vi "subVI PID.vi"(5 "PID gains":T1={"proportional gain (Kc)"=1.0, "integral time (Ti, s)"=0.01, "derivative time (Td, s)"=0.0} {"derivative time (Td, s)" format="%.3f"; "integral time (Ti, s)" format="%.3f"; "proportional gain (Kc)" format="%.3f"}, 6 "input":dbl, 7 "output range":cluster{"output high":dbl, "output low":dbl}={"output high"=100.0, "output low"=-100.0} {"output low" format="%.2f"; "output high" format="%.2f"}, 8 "reinitialize? (F)":bool, 9 "dt (s)":dbl=-1.0 format="%.3f", 10 "process variable":dbl format="%.2f", 11 "setpoint":dbl format="%.2f") -> (0 "dt out (s)":dbl format="%.3f", 3 "output":dbl format="%.2f")   [LabVIEW 2017]
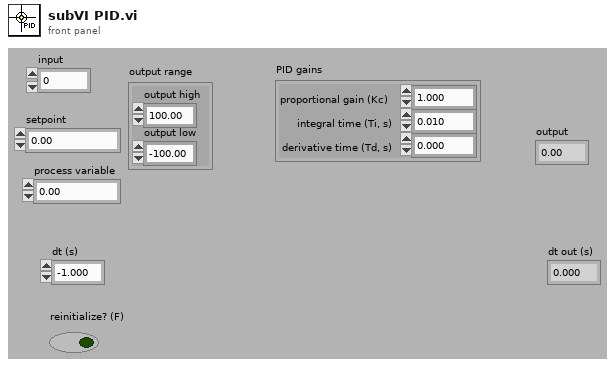
[diagram p1: front panel]
types:
  T1 = cluster{"proportional gain (Kc)":dbl, "integral time (Ti, s)":dbl, "derivative time (Td, s)":dbl}
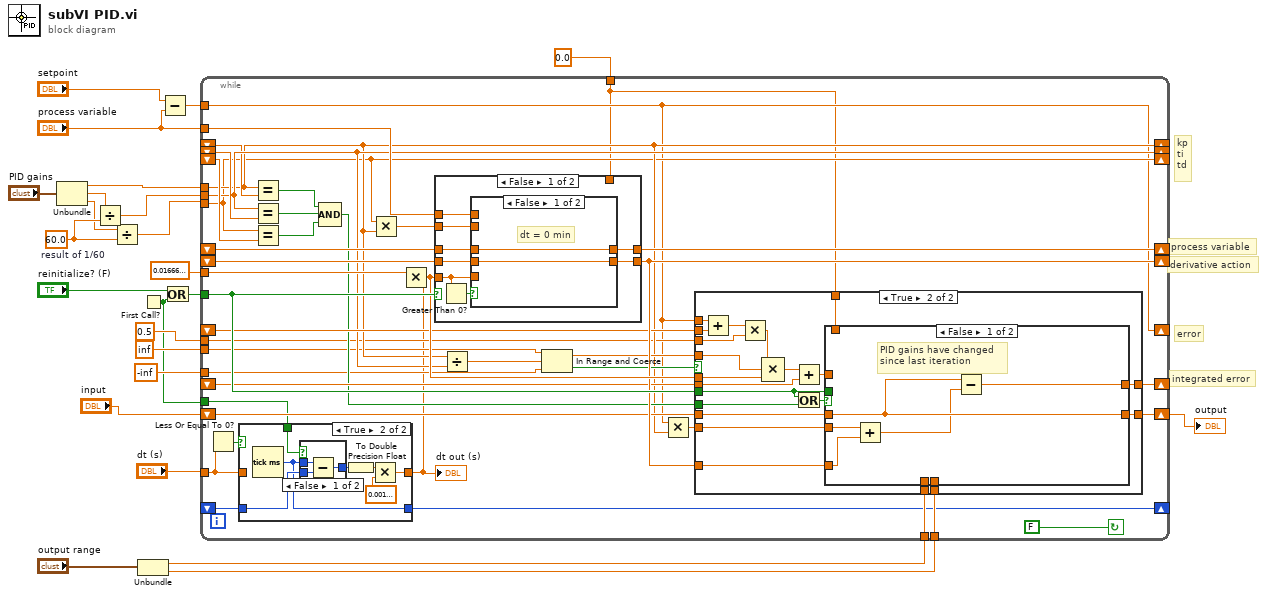
[diagram p0: block diagram]
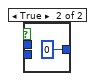
[diagram p3: hidden frame]
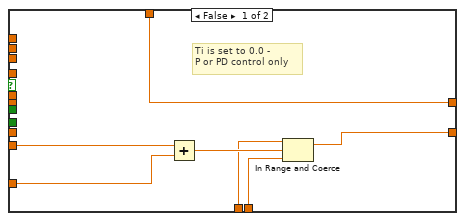
[diagram p4: hidden frame]
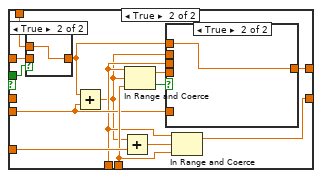
[diagram p5: hidden frame]
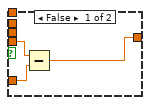
[diagram p6: hidden frame]
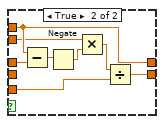
[diagram p8: hidden frame]
diagram:
  w6 = 60.0 ("y")
  w20 = 0.016666666666666666  # result of 1/60
  # "derivative action"
  # "process variable"
  # "kp\nti\ntd"
  # "error"
  # "integrated error"
  n1 = Unbundle("PID gains") -> ("proportional gain (Kc)"=w23:dbl, "integral time (Ti, s)"=w5:dbl, "derivative time (Td, s)"=w3:dbl)
  n2 = Divide(x=w5, y=w6) -> (x/y=w4:dbl)
  n3 = Divide(x=w3, y=w6) -> (x/y=w2:dbl)
  n4 = Unbundle("output range") -> ("output high"=w22:dbl, "output low"=w21:dbl)
  n5 = First Call?() -> (First Call?: T/F=w9:bool)
  n6 = Subtract(x="setpoint", y="process variable") -> (x-y=w11:dbl)
  n7 = Or(x="reinitialize? (F)", y=w9) -> (x .or. y?=w24:bool)
  n8 = while {
    tunnel: w24 -> [w66]
    shift-left: _ -> [w28]
    shift-right: [w29] -> _
    shift-right: [w38] -> _
    shift-left: _ -> [w39]
    shift-right: [w40] -> _
    shift-left: _ -> [w63]
    shift-right: [w33] -> _
    shift-left: _ -> [w64]
    tunnel: w23 -> [w38]
    tunnel: w4 -> [w40]
    tunnel: w2 -> [w33]
    tunnel: "dt (s)" -> [w27]
    tunnel: w22 -> [w59]
    tunnel: w21 -> [w58]
    tunnel: "process variable" -> [w57]
    shift-right: [w56] -> _
    shift-left: _ -> [w55]
    shift-right: [w54] -> _
    shift-left: _ -> [w46]
    shift-right: [w53] -> w13
    shift-left: "input" -> [w52]
    shift-right: [w32] -> _
    shift-left: _ -> [w51]
    shift-right: [w50] -> _
    shift-left: _ -> [w49]
    tunnel: w20 -> [w43]
    tunnel: 0.5 ("y") -> [w37]
    tunnel: inf ("upper limit") -> [w35]
    tunnel: -inf ("lower limit") -> [w36]
    tunnel: w11 -> [w32]
    tunnel: 0.0 -> [w31]
    tunnel: w9 -> [w25]
    stop <- FALSE continue-if-true
    n9 = Less Or Equal To 0?(x=w27) -> (x <= 0?=w26:bool)
    n10 = case shown="True" w26 {
      tunnel: [w68 w72] -> w30
      tunnel: w28 -> [w67 w71]
      tunnel: [w67 w70] -> w29
      tunnel: w27 -> [w68 _]
      tunnel: w25 -> [_ w69]
      frame False {
      }
      frame True {
        n11 = Tick Count (ms)() -> (millisecond timer value=w70:u32)
        n12 = case shown="False" w69 {
          tunnel: [w78 u32 0] -> w74
          tunnel: w71 -> [w77 _]
          tunnel: w70 -> [w76 _]
          frame False {
            n13 = Subtract(x=w76, y=w77) -> (x-y=w78:u32)
          }
          frame True {
          }
        }
        n14 = To Double Precision Float(number=w74) -> (double precision float=w73:dbl)
        n15 = Multiply(x=w73, y=0.0010000000474974513) -> (x*y=w72:dbl)
      }
    }
    "dt out (s)" <- w30
    n16 = Equal?(x=w38, y=w39) -> (x = y?=w61:bool)
    n17 = Equal?(x=w40, y=w63) -> (x = y?=w60:bool)
    n18 = Equal?(x=w33, y=w64) -> (x = y?=w62:bool)
    n19 = Compound Arithmetic op=AND(w61, w60, w62) -> (w41:bool)
    n20 = Multiply(x=w33, y=w38) -> (x*y=w45:dbl)
    n21 = Multiply(x=w43, y=w30) -> (x*y=w65:dbl)
    n22 = case shown="False" w66 {
      tunnel: w55 -> [w140 _]
      tunnel: w45 -> [w137 _]
      tunnel: w57 -> [w139 w152]
      tunnel: [w136 w152] -> w56
      tunnel: [w138 w151] -> w54
      tunnel: w46 -> [w134 _]
      tunnel: w65 -> [w133 _]
      tunnel: w31 -> [_ w151]
      frame False {
        n23 = Greater Than 0?(x=w133) -> (x > 0?=w135:bool)
        n24 = case shown="False" w135 {
          tunnel: w140 -> [w142 w148]
          tunnel: w133 -> [_ w147]
          tunnel: w139 -> [_ w145]
          tunnel: [w141 w146] -> w138
          tunnel: w137 -> [_ w143]
          tunnel: [w142 w145] -> w136
          tunnel: w134 -> [w141 _]
          frame False {
            # "dt = 0 min"
          }
          frame True {
            n25 = Subtract(x=w145, y=w148) -> (x-y=w150:dbl)
            n26 = Negate(x=w150) -> (-x=w144:dbl)
            n27 = Multiply(x=w143, y=w144) -> (x*y=w149:dbl)
            n28 = Divide(x=w149, y=w147) -> (x/y=w146:dbl)
          }
        }
      }
      frame True {
      }
    }
    n29 = Divide(x=w38, y=w40) -> (x/y=w44:dbl)
    n30 = In Range and Coerce(upper limit=w35, x=w44, lower limit=w36) -> (coerced(x)=w48:dbl, In Range?=w47:bool)
    n31 = Multiply(x=w32, y=w38) -> (x*y=w42:dbl)
    n32 = case shown="True" w47 {
      tunnel: w32 -> [_ w106]
      tunnel: w51 -> [_ w107]
      tunnel: w49 -> [_ w102]
      tunnel: [w80 w97] -> w50
      tunnel: w48 -> [_ w95]
      tunnel: w42 -> [w85 w100]
      tunnel: [w86 w96] -> w53
      tunnel: w52 -> [_ w98]
      tunnel: w54 -> [w84 w94]
      tunnel: w66 -> [_ w93]
      tunnel: w41 -> [_ w92]
      tunnel: w65 -> [_ w91]
      tunnel: w59 -> [w82 w89]
      tunnel: w58 -> [w81 w90]
      tunnel: w37 -> [_ w88]
      tunnel: w31 -> [w80 w87]
      frame False {
        # "Ti is set to 0.0 -\nP or PD control only"
        n33 = Add(x=w85, y=w84) -> (x+y=w83:dbl)
        n34 = In Range and Coerce(upper limit=w82, x=w83, lower limit=w81) -> (coerced(x)=w86:dbl)  [unwired: 1 out]
      }
      frame True {
        n35 = Add(x=w106, y=w107) -> (x+y=w105:dbl)
        n36 = Multiply(x=w105, y=w88) -> (x*y=w104:dbl)
        n37 = Compound Arithmetic op=MULTIPLY(w104, w95, w91) -> (w103:dbl)
        n38 = Add(x=w103, y=w102) -> (x+y=w101:dbl)
        n39 = Or(x=w93, y=w92) -> (x .or. y?=w99:bool)
        n40 = case shown="False" w99 {
          tunnel: w101 -> [_ w120]
          tunnel: w100 -> [w110 w115]
          tunnel: w98 -> [w112 _]
          tunnel: w93 -> [_ w122]
          tunnel: [w111 w117] -> w97
          tunnel: [w112 w125] -> w96
          tunnel: w94 -> [w109 w124]
          tunnel: w90 -> [_ w123]
          tunnel: w89 -> [_ w114]
          tunnel: w87 -> [_ w121]
          frame False {
            # "PID gains have changed\nsince last iteration"
            n41 = Add(x=w110, y=w109) -> (x+y=w108:dbl)
            n42 = Subtract(x=w112, y=w108) -> (x-y=w111:dbl)
          }
          frame True {
            n43 = case shown="True" w122 {
              tunnel: w121 -> [_ w132]
              tunnel: [w131 w132] -> w119
              tunnel: w120 -> [w131 _]
              frame False {
              }
              frame True {
              }
            }
            n44 = Add(x=w119, y=w115) -> (x+y=w113:dbl)
            n45 = Add(x=w113, y=w124) -> (x+y=w126:dbl)
            n46 = In Range and Coerce(upper limit=w114, x=w113, lower limit=w123) -> (coerced(x)=w116:dbl, In Range?=w118:bool)
            n47 = case shown="True" w118 {
              tunnel: w119 -> [_ w130]
              tunnel: [w127 w130] -> w117
              tunnel: w116 -> [w129 _]
              tunnel: w115 -> [w128 _]
              tunnel: w114 -> [_ _]
              tunnel: w113 -> [_ _]
              frame False {
                n48 = Subtract(x=w129, y=w128) -> (x-y=w127:dbl)
              }
              frame True {
              }
            }
            n49 = In Range and Coerce(upper limit=w114, x=w126, lower limit=w123) -> (coerced(x)=w125:dbl)  [unwired: 1 out]
          }
        }
      }
    }
  }
  "output" <- w13
